vi "SwapWithTblHist.vi"(7 "Table CtlRef In":refnum<vi>, 8 "error in (no error)":errorcluster, 9 "Mode Index":i32=2, 10 "Undo pointer":i32, 11 "OldTable Array in":T2) -> (0 "error out":errorcluster, 1 "changed? subarray":bool[][](array[boolean]), 2 "Change start":T1, 3 "OldTable Array out":T2, 4 "Mode change?":bool, 6 "Size mismatch?":bool)   [LabVIEW 2013]
doc: "Swap the present table value with a particular element in OldTable Array (history)."
uses:
  TypeDefs/TableArray.ctl
  <vilib>/Utility/miscctls.llb/LVRowAndColumnTypeDef.ctl
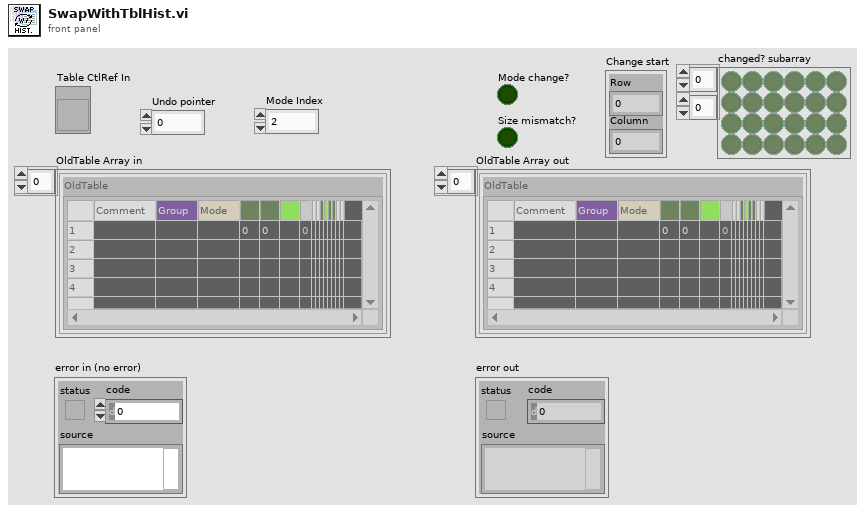
[diagram p1: front panel]
types:
  T1 = typedef "LVRowAndColumnTypeDef.ctl" = cluster{"Row":i32, "Column":i32}
  T2 = typedef "TableArray.ctl" = cluster{"OldTable":string[][]}[]
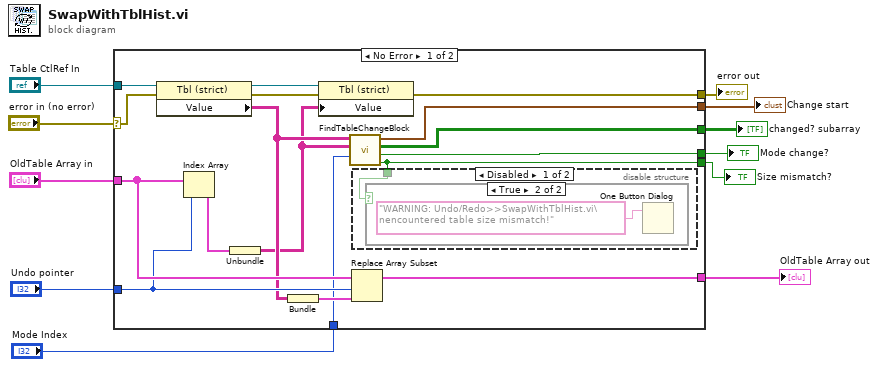
[diagram p0: block diagram]
diagram:
  n1 = case shown="No Error" "error in (no error)" {
    selector: "error in (no error)" -> [w19 w32]
    tunnel: "Table CtlRef In" -> [w26 _]
    tunnel: [w25 w32] -> w10
    tunnel: "OldTable Array in" -> [w24 w31]
    tunnel: "Undo pointer" -> [w23 _]
    tunnel: [w20 w31] -> w7
    tunnel: [w16 _] -> w5
    tunnel: [w15 _] -> w1
    tunnel: [w14 _] -> w4
    tunnel: "Mode Index" -> [w13 _]
    tunnel: [w12 _] -> w2
    frame No Error {
      n2 = property on="Property Node" class="Tbl (strict)"(reference=w26, error in=w19) -> (reference out=w28:refnum<vi>, error out=w27:errorcluster, "Value"=w18:string[][])
      n3 = Index Array "Index Array"(array=w24, index=w23) -> (element=w22:cluster{"OldTable":string[][]})
      n4 = Unbundle(w22) -> ("OldTable"=w17:string[][])
      n5 = Bundle("Value"=w18) -> (w21:cluster{"Value":string[][]})  [unwired: 1 in]
      n6 = property class="Tbl (strict)"(reference=w28, error in=w27, "Value"=w17) -> (error out=w25:errorcluster)  [unwired: 1 out]
      n7 = call "FindTableChangeBlock.vi"("Mode Index"=w13, "New Array"=w17, "Old Array"=w18) -> ("Size mismatch?"=w12:bool, "Mode change?"=w14:bool, "changed? subarray"=w15:bool[][], "Change start"=w16:T1)  [unwired: 5 in]
      n8 = Replace Array Subset "Replace Array Subset"(array=w24, new element=w21, index=w23) -> (w20:T2)
      n9 = disable-structure shown="Disabled" {
        disable-tunnel: w12 -> [w29 _]
        frame Disabled {
          n10 = case shown="True" w29 {
            frame False {
            }
            frame True {
              n11 = One Button Dialog(message="WARNING: Undo/Redo>>SwapWithTblHist.vi\nencountered table size mismatch!") -> ()  [unwired: 1 in, 1 out]
            }
          }
        }
        frame Enabled {
        }
      }
    }
    frame Error {
    }
  }
  "error out" <- w10
  "OldTable Array out" <- w7
  "Change start" <- w5
  "Mode change?" <- w4
  "Size mismatch?" <- w2
  "changed? subarray" <- w1
